vi "Create.vi"(5 "Grid Size":T1={"Width"=8, "Height"=8}, 7 "Clip Limit":dbl=2.0, 8 "error in (no error)":errorcluster) -> (0 "error out":errorcluster, 3 "CLAHE":refnum<class "CLAHE.lvclass">)   [LabVIEW 2020, in "image.lvlib" / "CLAHE.lvclass"]
doc: "CLAHE (Contrast Limited Adaptive Histogram Equalization)\n\nhttps://docs.opencv.org/4.11.0/d5/daf/tutorial_py_histogram_equalization.html"
uses:
  CLAHE.lvclass
  common/Image Size (Integer).ctl
  CLAHE.lvclass/CLAHE.ctl
  common/common.lvlib
  common/bin/gartoolkit_32-1.dll
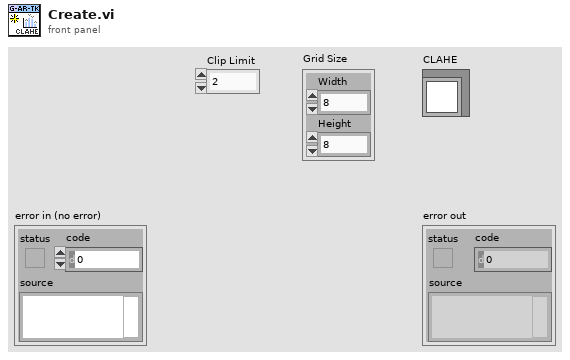
[diagram p1: front panel]
types:
  T1 = typedef "common.lvlib/Image Size (Integer).ctl" = cluster{"Width":u16, "Height":u16}
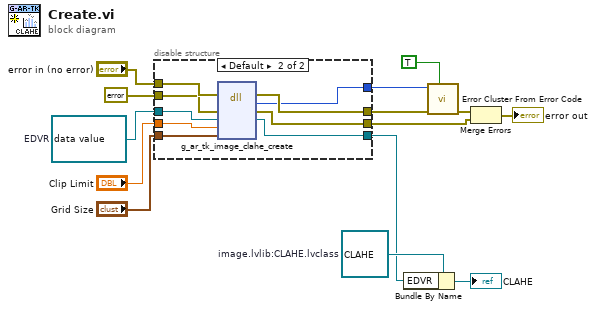
[diagram p0: block diagram]
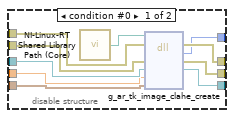
[diagram p2: hidden frame]
diagram:
  w3 = refnum<class "CLAHE.lvclass"> refnum  # image.lvlib:CLAHE.lvclass
  w12 = refnum<data-value> refnum  # EDVR
  n1 = disable-structure shown="Default" {
    disable-tunnel: "error in (no error)" -> [w23 w33]
    disable-tunnel: errorcluster {"status"=FALSE, "code"=0, "source"=""} ("error constant") -> [w24 w32]
    disable-tunnel: w12 -> [w21 w28]
    disable-tunnel: [w19 w31] -> w11
    disable-tunnel: [w17 w30] -> w10
    disable-tunnel: [w18 w29] -> w9
    disable-tunnel: "Clip Limit" -> [w20 w27]
    disable-tunnel: "Grid Size" -> [w15 w26]
    disable-tunnel: [w16 w25] -> w2
    frame condition #0 {
      n2 = call "NI-Linux-RT Shared Library Path (Core).vi"() -> ("Path"=w22:path)
      n3 = dll-call lib="?" fn="g_ar_tk_image_clahe_create" ("g_ar_toolkit.*.*:g_ar_tk_image_copy")(path in=w22, error in=w23, "error_cluster"=w24, "EDVR"=w21, "clip_limit"=w20, "grid_size"=w15) -> (error out=w19:errorcluster, "return type"=w17:i32, "error_cluster"=w18:errorcluster, "EDVR"=w16:refnum<data-value>)  [unwired: 3 in, 1 out]
    }
    frame condition #1 (active) {
      n4 = dll-call lib="C:/serenial/lib/g-augmented-reality-toolkit/LabVIEW/common/bin/gartoolkit_*-1.*" fn="g_ar_tk_image_clahe_create" ("g_ar_toolkit.*.*:g_ar_tk_image_copy")(error in=w33, "error_cluster"=w32, "EDVR"=w28, "clip_limit"=w27, "grid_size"=w26) -> (error out=w31:errorcluster, "return type"=w30:i32, "error_cluster"=w29:errorcluster, "EDVR"=w25:refnum<data-value>)  [unwired: 4 in, 1 out]
    }
  }
  n5 = Bundle By Name(cluster=w3, "EDVR"=w2) -> (→"CLAHE":refnum<class "CLAHE.lvclass">)
  n6 = call <vilib>:"Error Cluster From Error Code.vi"("show call chain? (False)"=TRUE, "error in (no error)"=w11, "error code (0)"=w10) -> ("error out"=w14:errorcluster)  [unwired: 6 in]
  n7 = Merge Errors(w14, w9) -> (→"error out":errorcluster)
